vi "Write Vector Network Analyzer.lvclass.vi"(10 "Vector Network Analyzer.lvclass":refnum<class "Vector Network Analyzer.lvclass">, 11 "PathControl in":refnum<class "PathControl.lvclass">) -> (3 "PathControl out":refnum<class "PathControl.lvclass">)   [LabVIEW 2020, in "PathControl.lvclass"]
uses:
  PathControl.lvclass
  Instruments/Vector Network Analyzer/Vector Network Analyzer.lvclass
  PathControl.lvclass/PathControl.ctl
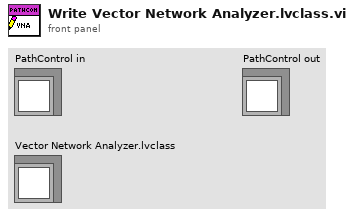
[diagram p1: front panel]
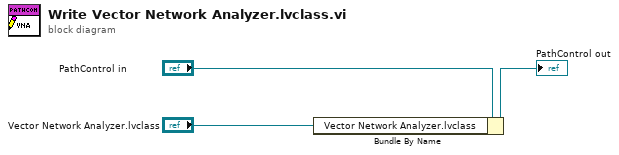
[diagram p0: block diagram]
diagram:
  n1 = Bundle By Name(cluster="PathControl in", "Vector Network Analyzer.lvclass"="Vector Network Analyzer.lvclass") -> (→"PathControl out":refnum<class "PathControl.lvclass">)
